vi "MikeTX.vi"() -> ()   [LabVIEW 2013]
uses:
  <vilib>/addons/Modulation/Digital/General/MT Generate Bits (Galois, PN Order).vi
  <vilib>/Analysis/2dsp.llb/Real FFT.vi
  <vilib>/addons/Modulation/Analog/support/mod_Set Error Source.vi
  <vilib>/addons/Modulation/Digital/Support/Common/Validators/mod_Generate Bits Validate.vi
  <vilib>/addons/Modulation/Digital/General/MT Apply Matched Filter (Generic).vi
  <vilib>/addons/Modulation/Digital/Support/Common/Validators/mod_Generate Filter Coefficients Validate.vi
  <vilib>/addons/Modulation/Digital/General/subVIs/mod_Generate Filter Coefficients.vi
  <instrlib>/niUSRP/niUSRP Write Tx Data (CDB).vi
  <vilib>/imath/engines/lvmath2/RunTimeEngine/ErrorHandling/NIMS_Finalize Error.vi
  <vilib>/imath/engines/lvmath2/RunTimeEngine/Managers/WorkSpace/UID Generator.vi
  <vilib>/imath/engines/lvmath2/RunTimeEngine/Managers/SymbolTable/Clear UID.vi
  <vilib>/imath/engines/lvmath2/RunTimeEngine/NodeEndStatement/NIMS_NodeEndStatement_Output.vi
  <instcachedir>/0/NIMS_NodeEndStatement_Output_53EC0D466D134D7ABD903AC30B43404B.lvgen/NIMS_NodeEndStatement_Output_53EC0D466D134D7ABD903AC30B43404B_002.vi
  <instcachedir>/0/NIMS_NodeEndStatement_Output_53EC0D466D134D7ABD903AC30B43404B.lvgen/NIMS_NodeEndStatement_Output_53EC0D466D134D7ABD903AC30B43404B_004.vi
  <vilib>/imath/engines/lvmath2/RunTimeEngine/BuiltInFunctions/buffermx/NIMS_[1o]_buffermx(V,I32).vi
  <instcachedir>/0/NIMS_[1o]_buffermx(V,I32)_B3D794E02CD04108991C55A1494CB1AE.lvgen/NIMS_[1o]_buffermx(V,I32)_B3D794E02CD04108991C55A1494CB1AE_000.vi
  <vilib>/imath/engines/lvmath2/RunTimeEngine/RunTimeType/NIMS_RunTimeType_From StrictType (excl LVString).vi
  <instcachedir>/0/NIMS_RunTimeType_From StrictType (excl LVString)_4DEE718D6EB74582AA20236969C084FC.lvgen/NIMS_RunTimeType_From StrictType (excl LVString)_4DEE718D6EB74582AA20236969C084FC_000.vi
  <vilib>/imath/engines/lvmath2/RunTimeEngine/LocalVariableDefStatement/MC_LocalVariableDefStatement_Display.vi
  <vilib>/imathl/engines/lvmath/Functions/Error Handling/Create Error.vi
  <vilib>/addons/Modulation/Digital/General/subVIs/mod_Generate Bits PN Sequence.vi
  <vilib>/Analysis/NI_AALBase.lvlib
  <vilib>/Analysis/NI_AALPro.lvlib
  <vilib>/addons/Modulation/niDMT.lvlib
  <vilib>/imath/engines/lvmath2/RunTimeEngine/Managers/SymbolTable/NIMS_WorkSpace.lvlib
panel:
  out "b":dbl
  out "a":dbl
  out "Waveform Graph 3":cluster{"t0":dbl, "dt":dbl, "Y":dbl[]}(graph)
  out "Waveform Graph 2":cluster{"t0":dbl, "dt":dbl, "Y":dbl[]}(graph)
  out "mathscript output":i32[](array[numeric])
  out "c output":dbl
  out "XY Graph 4":cdb[](graph)
  out "Es befor matched filter":ext
  out "XY Graph 3":cdb[](graph)
  out "XY Graph":cdb[](graph)
  out "Es":dbl
  out "energy before matched filter":dbl
  out "Discrete energy after matched filter":dbl
  out "Avg discrete power after matched filtering":dbl
  out "symbols":ext
  out "# pulse filter taps":i32
  out "energy of pulse":dbl
  out "I and Q aftre matched fltering, before sampling":cdb[](graph) caption="hata allt, framför allt labview"
  in  "PN sequence order (15)":i32=9
  in  "reset phase 2":bool=TRUE
  in  "samples 2":i32=128
  in  "frequency 4":dbl=0.0078125 format="%0.4e"
  in  "reset phase":bool=TRUE
  in  "carrier frequency":dbl=100000.0 format="%#_6p"
  in  "samples":i32=128
  in  "frequency 3":dbl=0.0078125 format="%0.4e"
  in  "channel list":string
  out "Waveform Graph":dbl[](graph)
  in  "stop":bool
  out "coerced gain":dbl format="%#_6f"
  out "coerced IQ rate":dbl=100000.0 format="%#_6p"
  in  "active antenna":string
  in  "gain":dbl format="%#_6f"
  in  "IQ rate":dbl=100000.0 format="%#_6p"
  in  "device names":refnum<k15>
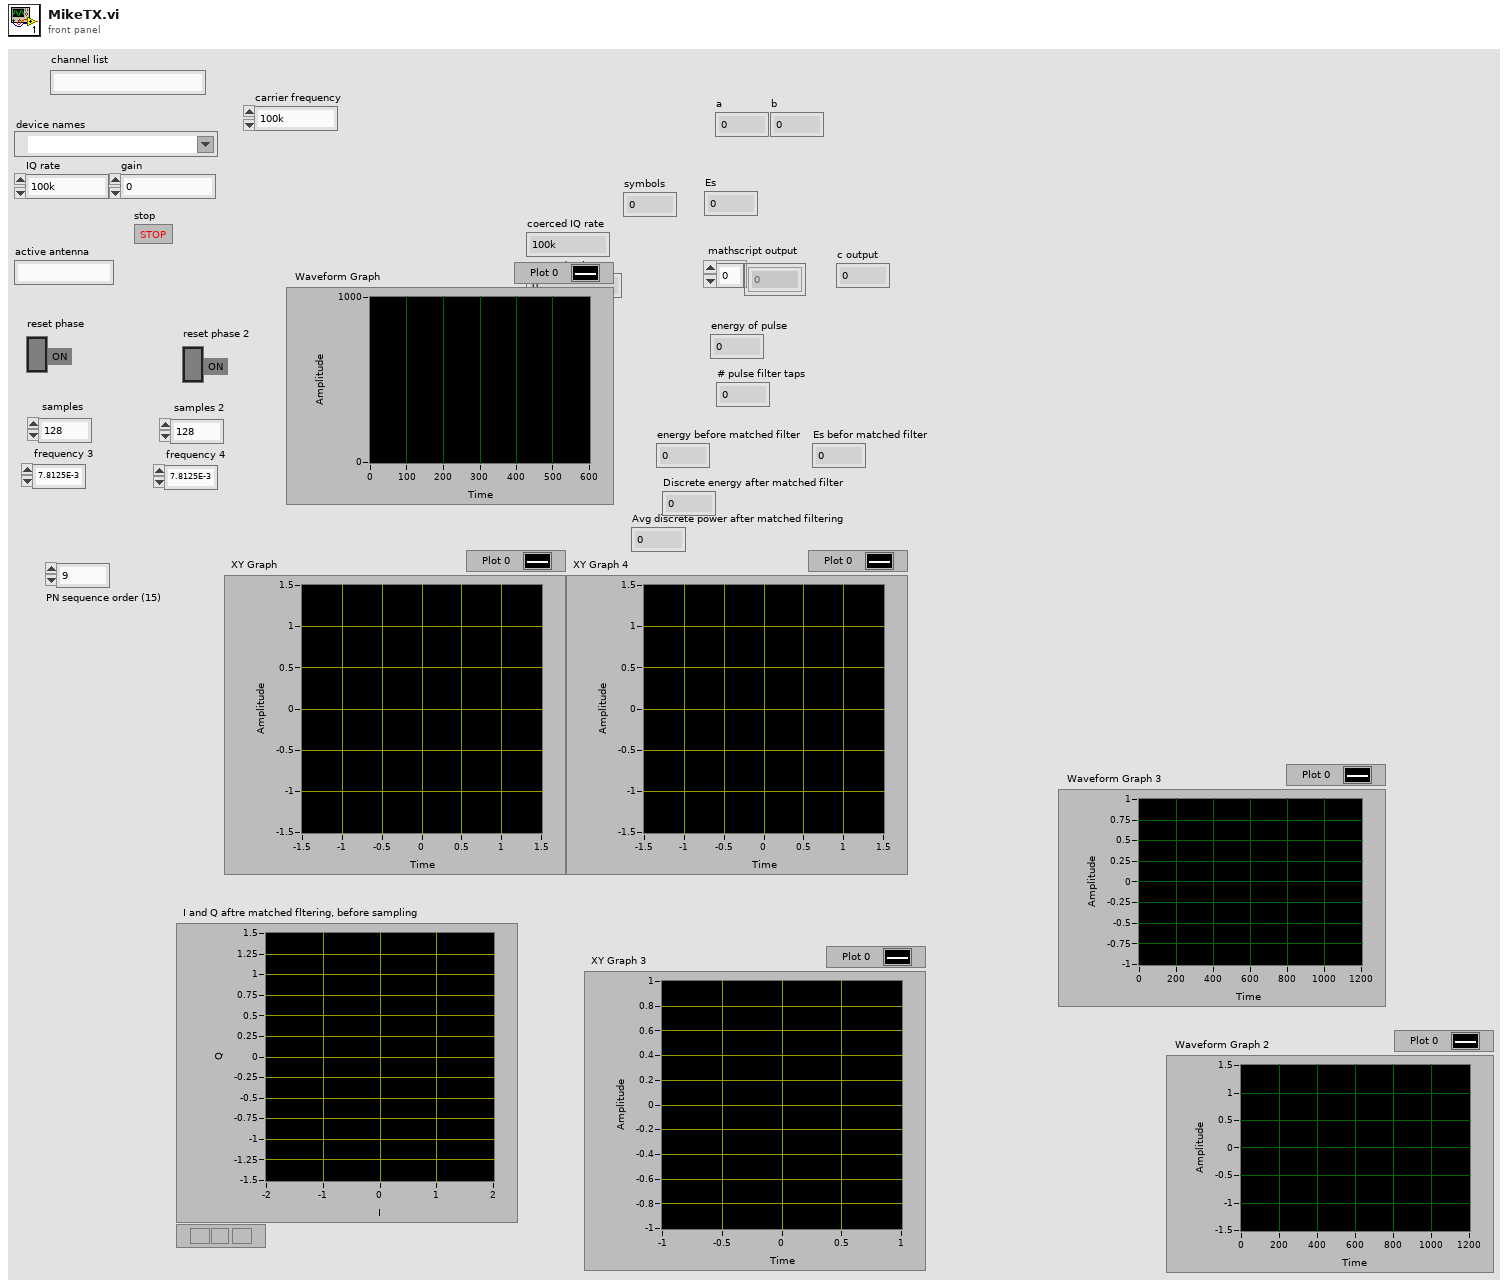
[diagram p1: front panel]
types:
  T1 = enum16{"none", "Raised Cosine", "Root Raised Cos", "Gaussian"}
  T2 = enum16{"FSK", "PSK", "QAM", "MSK", "PAM", "ASK", "CPM"}
  T3 = cluster{"samples per symbol (16)":i32, "symbol map":cdb[]}
  T4 = typedef "niAMT.lvlib/Complex Data Waveform.ctl" = cluster{"t0":dbl, "dt":dbl, "Y":cdb[]}
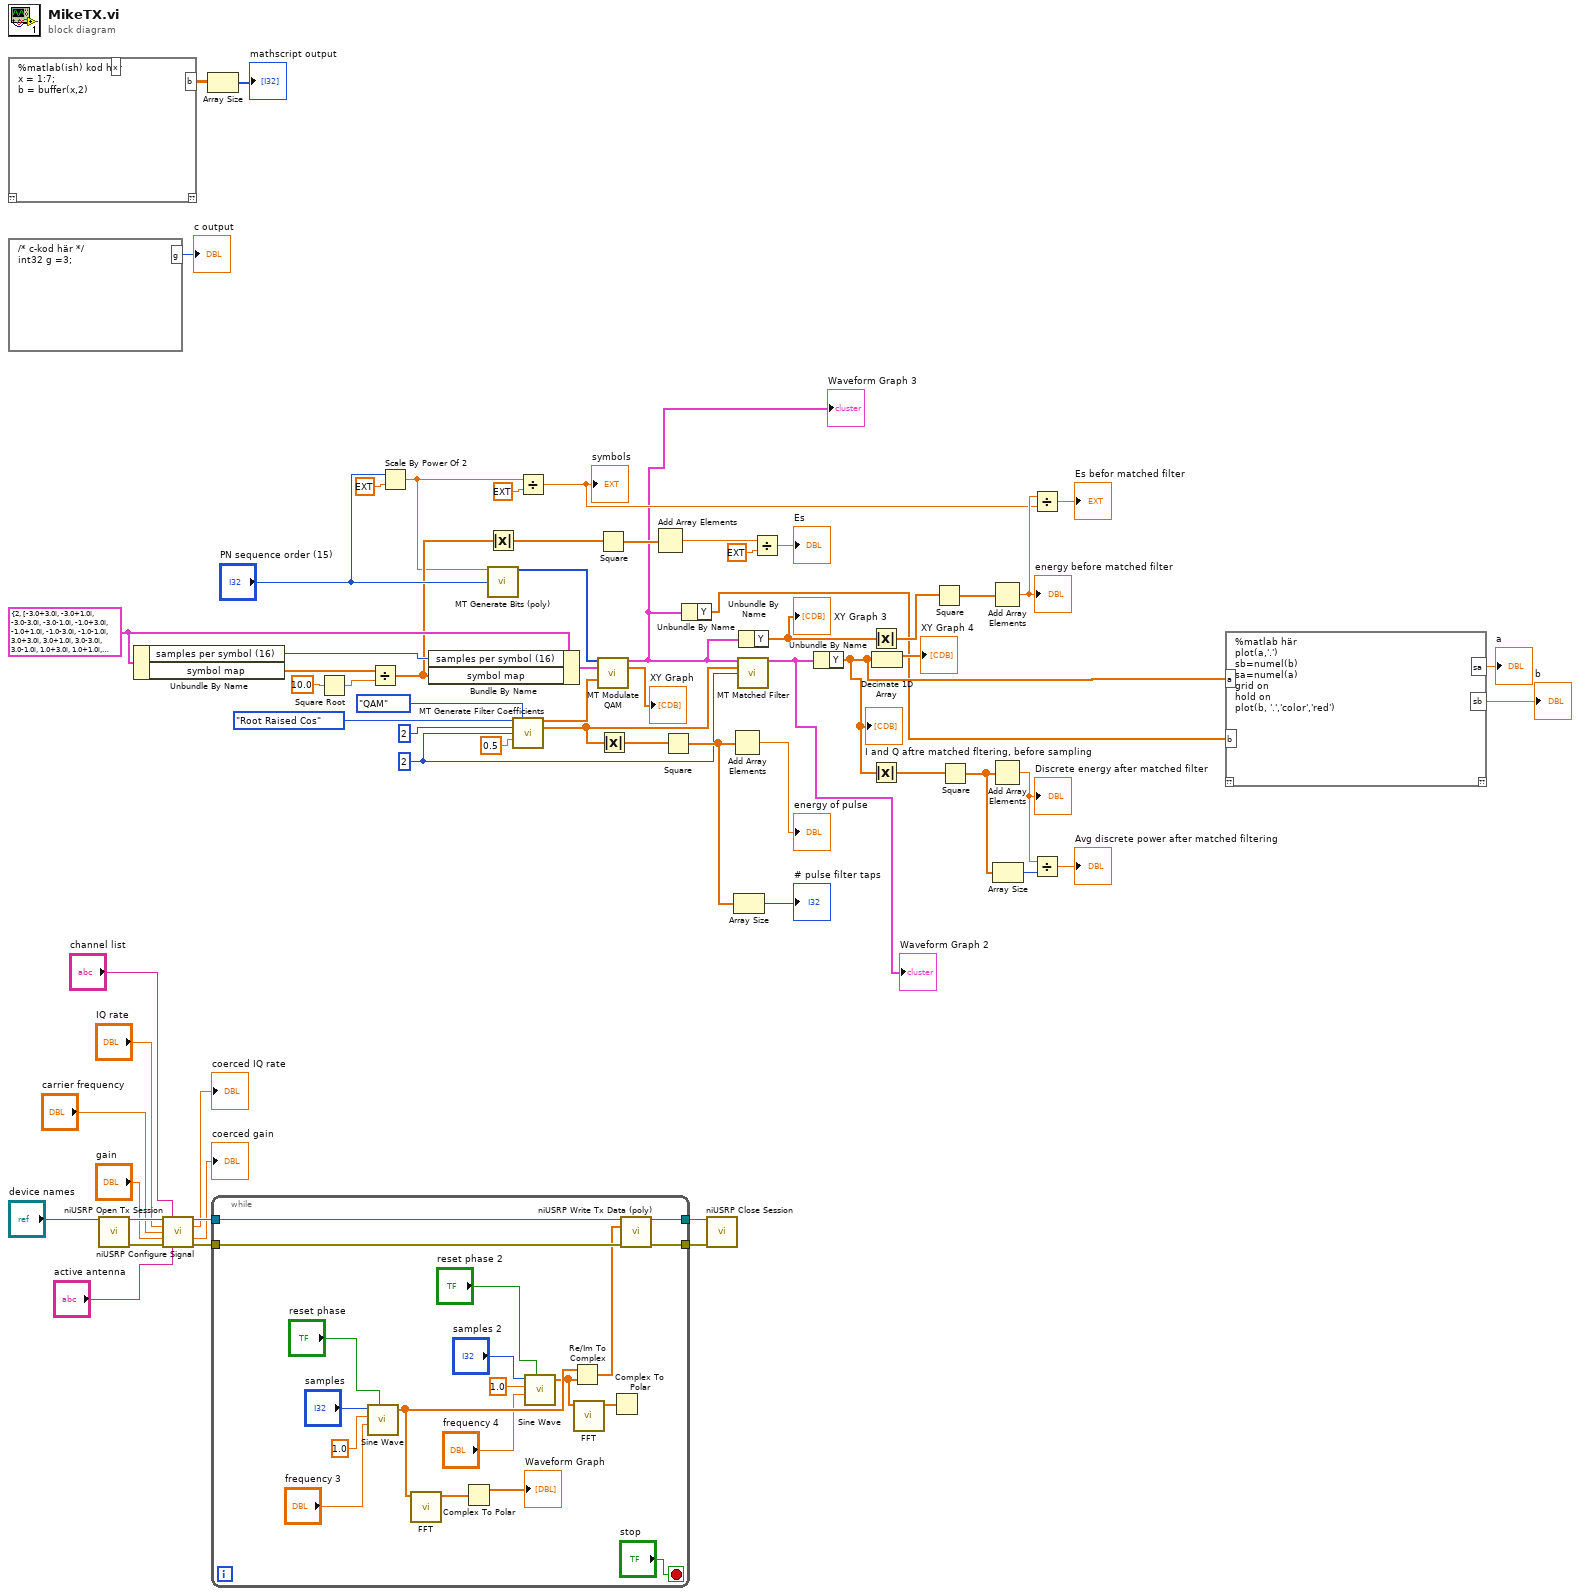
[diagram p0: block diagram]
diagram:
  w13 = 2 ("pulse shaping samples per symbol (16)")
  w30 = T3 {"samples per symbol (16)"=2, "symbol map"=[-3.0+3.0i, -3.0+1.0i, -3.0-3.0i, -3.0-1.0i, -1.0+3.0i, -1.0+1.0i, -1.0-3.0i, -1.0-1.0i, 3.0+3.0i, 3.0+1.0i, 3.0-3.0i, 3.0-1.0i, 1.0+3.0i, 1.0+1.0i, 1.0-3.0i, 1.0-1.0i]} ("QAM system parameters")
  n1 = mathscript code="%matlab(ish) kod här \nx = 1:7;\nb = buffer(x,2)"() -> ("b"=w10:dbl[][])  [unwired: 1 in, 2 out]
  n2 = formula code="/* c-kod här */\nint32 g =3;"() -> ("g"=→"c output":i32)
  n3 = call <instrlib>:"niUSRP Open Tx Session.vi"("device names"="device names") -> ("session handle out"=w64:refnum<k15>, "error out"=w63:errorcluster)  [unwired: 13 in]
  n4 = Unbundle By Name(w30) -> ("samples per symbol (16)"=w34:i32, "symbol map"=w31:cdb[])
  n5 = call <instrlib>:"niUSRP Configure Signal.vi"("session handle"=w64, "channel list"="channel list", "IQ rate"="IQ rate", "carrier frequency"="carrier frequency", "gain"="gain", "error in (no error)"=w63, "active antenna"="active antenna") -> ("session handle out"=w62:refnum<k15>, "coerced IQ rate"=→"coerced IQ rate":dbl, "coerced gain"=→"coerced gain":dbl, "error out"=w61:errorcluster)  [unwired: 4 in, 1 out]
  n6 = Array Size(array=w10) -> (size(s)=→"mathscript output":i32[])
  n7 = while {
    tunnel: w62 -> [w83]
    tunnel: w61 -> [w82]
    tunnel: [w81] -> w60
    tunnel: [w80] -> w59
    stop <- "stop" stop-if-true
    n8 = call <vilib>:"Sine Wave.vi"("samples"="samples", "amplitude"=1.0, "frequency"="frequency 3", "reset phase"="reset phase") -> ("sine wave"=w75:dbl[])  [unwired: 1 in, 2 out]
    n9 = call-poly <vilib>:"FFT.vi"("X"=w75) -> ("FFT {X}"=w78:cdb[])  [unwired: 9 in, 1 out]
    n10 = Complex To Polar(r * e^(i*theta)=w78) -> (r=→"Waveform Graph":dbl[])  [unwired: 1 out]
    n11 = call <vilib>:"Sine Wave.vi"("samples"="samples 2", "amplitude"=1.0, "frequency"="frequency 4", "reset phase"="reset phase 2") -> ("sine wave"=w65:dbl[])  [unwired: 1 in, 2 out]
    n12 = Re/Im To Complex(1:w65, 2:w75) -> (0:w74:cdb[])
    n13 = call-poly <vilib>:"FFT.vi"("X"=w65) -> ("FFT {X}"=w76:cdb[])  [unwired: 9 in, 1 out]
    n14 = Complex To Polar(r * e^(i*theta)=w76) -> ()  [unwired: 2 out]
    n15 = call-poly <instrlib>:"niUSRP Write Tx Data (poly).vi"("session handle"=w83, "data"=w74, "error in (no error)"=w82) -> ("session handle out"=w81:refnum<k15>, "error out"=w80:errorcluster)  [unwired: 11 in]
  }
  n16 = Square Root(x=10.0 ("y")) -> (sqrt(x)=w32:dbl)
  n17 = Divide(x=w31, y=w32) -> (x/y=w26:cdb[])
  n18 = Scale By Power Of 2(n="PN sequence order (15)", x=ext 1.0) -> (x*2^n=w16:ext)
  n19 = Bundle By Name(cluster=w30, "samples per symbol (16)"=w34, "symbol map"=w26) -> (w29:T3)
  n20 = Absolute Value(x=w26) -> (abs(x)=w28:dbl[])
  n21 = call-poly <vilib>:"MT Generate Bits (poly).vi"("total bits (128)"=w16, "PN sequence order (9)"="PN sequence order (15)") -> ("output bit stream"=w48:i8[])  [unwired: 11 in, 2 out]
  n22 = call <vilib>:"MT Generate Filter Coefficients.vi"("pulse shaping filter (none)"=T1."Root Raised Cos", "modulation type"=T2."QAM", "pulse shaping samples per symbol (16)"=2, "matched samples per symbol (16)"=w13, "filter parameter"=0.5) -> ("pulse shaping filter coefficients"=w46:dbl[], "matched filter coefficients"=w40:dbl[])  [unwired: 8 in, 1 out]
  n23 = Divide(x=w16, y=ext 4.0) -> (x/y=w15:ext)
  "symbols" <- w15
  n24 = Square(x=w28) -> (x^2=w27:dbl[])
  n25 = call <vilib>:"MT Modulate QAM.vi"("input bit stream"=w48, "QAM system parameters"=w29, "pulse shaping filter coefficients"=w46) -> ("output complex waveform"=w2:T4, "symbols out"=→"XY Graph":cdb[])  [unwired: 10 in, 1 out]
  "Waveform Graph 3" <- w2
  n26 = Absolute Value(x=w40) -> (abs(x)=w43:dbl[])
  n27 = Add Array Elements(numeric array=w27) -> (sum=w24:dbl)
  n28 = Square(x=w43) -> (x^2=w42:dbl[])
  n29 = Unbundle By Name(w2) -> ("Y"=w1:cdb[])
  n30 = call <instrlib>:"niUSRP Close Session.vi"("session handle"=w60, "error in (no error)"=w59) -> ()  [unwired: 13 in, 1 out]
  n31 = Add Array Elements(numeric array=w42) -> (sum=→"energy of pulse":dbl)
  n32 = Array Size(array=w42) -> (size(s)=→"# pulse filter taps":i32)
  n33 = call-poly <vilib>:"MT Matched Filter.vi"("input complex waveform"=w2, "matched filter coefficients"=w40, "samples per symbol (16)"=w13) -> ("output complex waveform"=w8:T4)  [unwired: 11 in, 1 out]
  "Waveform Graph 2" <- w8
  n34 = Unbundle By Name(w2) -> ("Y"=w22:cdb[])
  "XY Graph 3" <- w22
  n35 = Divide(x=w24, y=ext 16.0) -> (x/y=→"Es":ext)
  n36 = Unbundle By Name(w8) -> ("Y"=w5:cdb[])
  "I and Q aftre matched fltering, before sampling" <- w5
  n37 = Absolute Value(x=w22) -> (abs(x)=w36:dbl[])
  n38 = Absolute Value(x=w5) -> (abs(x)=w44:dbl[])
  n39 = Decimate 1D Array(w5) -> (→"XY Graph 4":cdb[])  [unwired: 1 out]
  n40 = Square(x=w36) -> (x^2=w19:dbl[])
  n41 = Square(x=w44) -> (x^2=w21:dbl[])
  n42 = Add Array Elements(numeric array=w19) -> (sum=w18:dbl)
  "energy before matched filter" <- w18
  n43 = Add Array Elements(numeric array=w21) -> (sum=w37:dbl)
  "Discrete energy after matched filter" <- w37
  n44 = Array Size(array=w21) -> (size(s)=w20:i32)
  n45 = Divide(x=w18, y=w15) -> (x/y=→"Es befor matched filter":ext)
  n46 = Divide(x=w37, y=w20) -> (x/y=→"Avg discrete power after matched filtering":dbl)
  n47 = script code="%matlab här\nplot(a,'.')\nsb=numel(b)\nsa=numel(a)\ngrid on\nhold on\nplot(b, '.','color','red')"("a"=w5, "b"=w1) -> ("sa"=→"a":dbl, "sb"=→"b":dbl)  [unwired: 1 in, 1 out]
